vi "Python Dialog.vi"() -> ()   [LabVIEW 2024]
panel:
  out "success":bool
  in  "test":bool
  in  "Update":bool
  in  "Python path":path
  in  "Python version":string="3.10"
  # "Settings"
  # "Please make sure both settings are correct\nand that you have run pip install bleak"
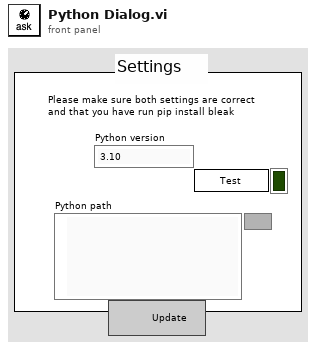
[diagram p1: front panel]
types:
  T1 = cluster{"Python version":string, "Python path":string}
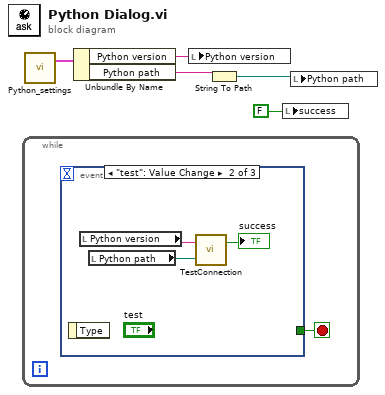
[diagram p0: block diagram]
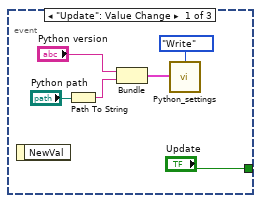
[diagram p2: hidden frame]
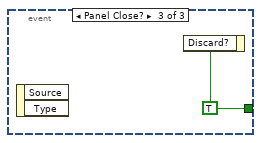
[diagram p3: hidden frame]
diagram:
  n1 = while {
    stop <- w6 stop-if-true
    n2 = event shown="[1] \"test\": Value Change" {
      selector: _ -> [_ _ _]
      dyn-events: _ -> [_ _ _]
      timeout: _ -> [_ _ _]
      tunnel: ["Update" _ w16] -> w6
      event "Update": Value Change {
        n3 = event-data() -> ()  [unwired: 1 in, 1 out]
        n4 = Path To String(path="Python path") -> (string=w11:string)
        n5 = Bundle("Python version"="Python version", w11) -> (w9:cluster{"Python version":string, string})  [unwired: 1 in]
        n6 = call "Python_settings.vi"("Task"=enum16{"Read", "Write"}."Write", "Settings in"=w9) -> ()  [unwired: 3 in, 1 out]
      }
      event "test": Value Change {
        n7 = event-data() -> ()  [unwired: 1 in, 1 out]
        n8 = local read "Python version"() -> (w15:string)
        n9 = local read "Python path"() -> (w14:path)
        n10 = call "TestConnection.vi"("Python path"=w14, "Python version"=w15) -> ("success?"=→"success":bool)  [unwired: 1 out]
      }
      event Panel Close? {
        w16 = TRUE
        n11 = event-data() -> ()  [unwired: 1 in, 2 out]
        n12 = event-data("Discard?"=w16) -> ()  [unwired: 1 in, 1 out]
      }
    }
  }
  n13 = call "Python_settings.vi"() -> ("settings read"=w5:T1)  [unwired: 5 in]
  n14 = Unbundle By Name(w5) -> ("Python version"=w4:string, "Python path"=w3:string)
  n15 = local write "Python version"(w4) -> ()
  n16 = String To Path(string=w3) -> (path=w2:path)
  n17 = local write "success"(FALSE ("success")) -> ()
  n18 = local write "Python path"(w2) -> ()
